vi "get child class link.vi"(8 "error in (no error)":errorcluster, 11 "node in":refnum<k20>) -> (0 "error out":errorcluster, 2 "link":string, 3 "node out":refnum<k20>)   [LabVIEW 2023]
uses:
  <resource>/objmgr/DOMUserDefRef.rc
  <vilib>/xml/NI_XML.lvlib
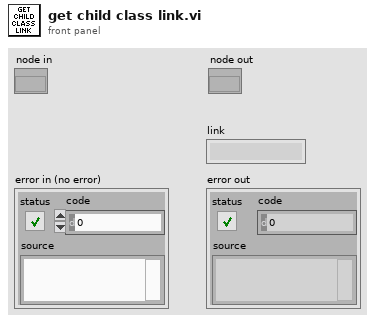
[diagram p1: front panel]
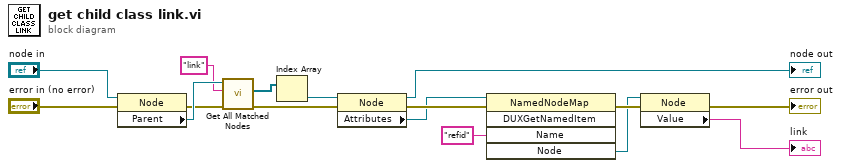
[diagram p0: block diagram]
diagram:
  n1 = property class="Node"(reference="node in", error in="error in (no error)") -> (error out=w10:errorcluster, "Parent"=w12:refnum<k20>)  [unwired: 1 out]
  n2 = call <vilib>:"Get All Matched Nodes.vi"("error in (no error)"=w10, "XPath expression"="link", "node in"=w12) -> ("error out"=w11:errorcluster, "node result array"=w13:refnum<k20>[])  [unwired: 6 in, 1 out]
  n3 = Index Array(array=w13) -> (element=w14:refnum<k20>)  [unwired: 1 in]
  n4 = property class="Node"(reference=w14, error in=w11) -> (reference out=→"node out":refnum<k20>, error out=w15:errorcluster, "Attributes"=w5:refnum<k20>)
  n5 = invoke class="NamedNodeMap" method="DUXGetNamedItem"(reference=w5, error in=w15, "Name"="refid") -> (error out=w8:errorcluster, "Node"=w7:refnum<k20>)  [unwired: 2 in, 3 out]
  n6 = property class="Node"(reference=w7, error in=w8) -> (error out=→"error out":errorcluster, "Value"=→"link":string)  [unwired: 1 out]
